vi "Read STEP N°.vi"(11 "STEP in":refnum<class "STEP.lvclass">) -> (2 "STEP N°":u32, 3 "STEP out":refnum<class "STEP.lvclass">)   [LabVIEW 2014, in "SeqLoop.lvlib" / "STEP Classes.lvlib" / "STEP.lvclass"]
uses:
  STEP.lvclass
  STEP.lvclass/STEP.ctl
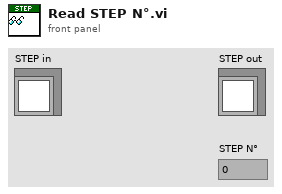
[diagram p1: front panel]
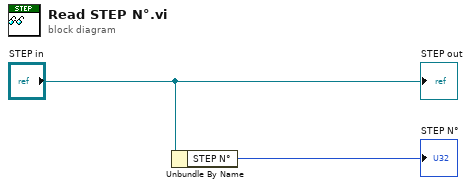
[diagram p0: block diagram]
diagram:
  n1 = Unbundle By Name("STEP in") -> ("STEP N°"=→"STEP N°":u32)
  "STEP out" <- "STEP in"
